vi "Compra.vi"(8 "error in (no error)":errorcluster, 10 "Producto":string[](array[string]), 11 "UI Actor in":refnum<class "UI Actor.lvclass">) -> (0 "error out":errorcluster, 3 "UI Actor out":refnum<class "UI Actor.lvclass">)   [LabVIEW 2019, in "UI Actor.lvlib" / "UI Actor.lvclass"]
uses:
  UI Actor.lvclass
  C:/Program Files/National Instruments/LabVIEW 2019/vi.lib/ActorFramework/Actor/Actor.lvclass
  <vilib>/ActorFramework/Actor/Actor.lvclass/Actor.ctl
  <vilib>/ActorFramework/Message Enqueuer/Message Enqueuer.lvclass/Message Enqueuer.ctl
  UI Actor.lvclass/UI Actor.ctl
  UI Actor Messages/Credit Update Coins Msg/Credit Update Coins Msg.lvclass/Credit Update Coins Msg.ctl
  <vilib>/ActorFramework/Message Enqueuer/Init from Existing Queue.vi
  <vilib>/ActorFramework/Message Enqueuer/Enqueue.vi
  UI Actor Messages/Credit Update Coins Msg/Credit Update Coins Msg.lvclass
  C:/Program Files/National Instruments/LabVIEW 2019/vi.lib/ActorFramework/Message/Message.lvclass
  <vilib>/ActorFramework/Message Priority Queue/Priority Enqueue.vi
  <vilib>/ActorFramework/Message Enqueuer/Message Enqueuer.lvclass
  <vilib>/ActorFramework/Actor/Actor.lvclass
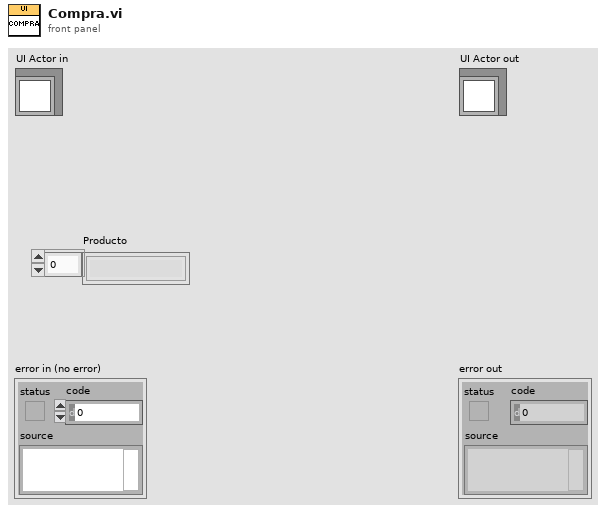
[diagram p1: front panel]
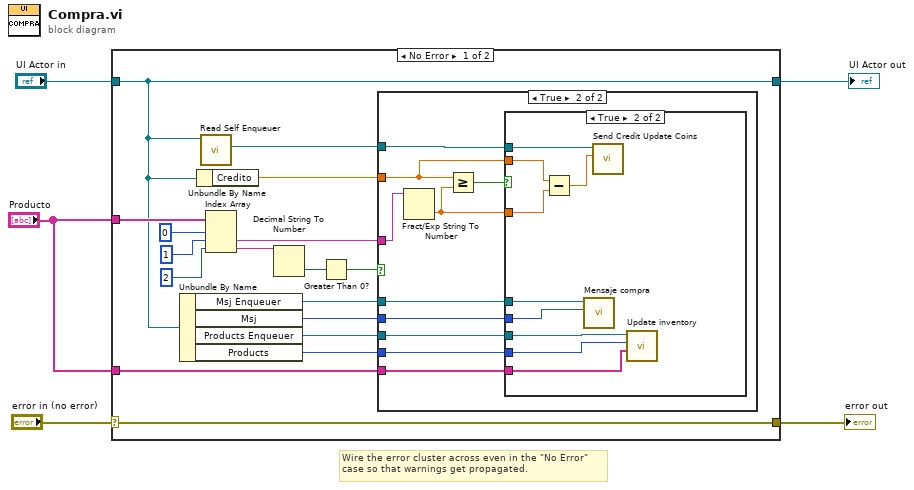
[diagram p0: block diagram]
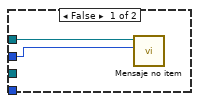
[diagram p2: hidden frame]
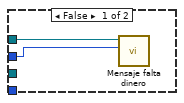
[diagram p3: hidden frame]
diagram:
  # "Wire the error cluster across even in the \"No Error\"\ncase so that warnings get propagated."
  n1 = case shown="No Error" "error in (no error)" {
    selector: "error in (no error)" -> [w22 w47]
    tunnel: [w22 w47] -> w4
    tunnel: [w8 w46] -> w2
    tunnel: "UI Actor in" -> [w8 w46]
    tunnel: "Producto" -> [w21 _]
    tunnel: "Producto" -> [w12 _]
    frame No Error {
      n2 = Unbundle By Name(w8) -> ("Msj Enqueuer"=w6:refnum<class "Message Enqueuer.lvclass">, "Msj"=w7:enum16{"ESP", "ING"}, "Products Enqueuer"=w10:refnum<class "Message Enqueuer.lvclass">, "Products"=w11:enum16{"Bakery", "Coffee"})
      n3 = Unbundle By Name(w8) -> ("Credito"=w14:dbl)
      n4 = call <vilib>:"Read Self Enqueuer.vi"("Actor"=w8) -> ("Self Enqueuer"=w9:refnum<class "Message Enqueuer.lvclass">)  [unwired: 10 in]
      n5 = Index Array(array=w21, index #1=0 ("index"), index #2=1 ("index"), index #3=2 ("index")) -> (element #2=w13:string, element #3=w17:string)  [unwired: 1 out]
      n6 = Decimal String To Number(string=w17) -> (number=w16:i32)  [unwired: 2 in, 1 out]
      n7 = Greater Than 0?(x=w16) -> (x > 0?=w15:bool)
      n8 = case shown="True" w15 {
        tunnel: w14 -> [_ w29]
        tunnel: w13 -> [_ w34]
        tunnel: w12 -> [_ w32]
        tunnel: w11 -> [_ w31]
        tunnel: w10 -> [_ w30]
        tunnel: w9 -> [_ w27]
        tunnel: w7 -> [w24 w26]
        tunnel: w6 -> [w23 w25]
        frame False {
          n9 = call "Mensaje no item.vi"("Msj"=w24, "Message Enqueuer in"=w23) -> ()  [unwired: 10 in]
        }
        frame True {
          n10 = Fract/Exp String To Number(string=w34) -> (number=w28:dbl)  [unwired: 3 in, 1 out]
          n11 = Greater Or Equal?(x=w29, y=w28) -> (x >= y?=w33:bool)
          n12 = case shown="True" w33 {
            tunnel: w32 -> [_ w45]
            tunnel: w31 -> [_ w44]
            tunnel: w30 -> [_ w43]
            tunnel: w29 -> [_ w42]
            tunnel: w28 -> [_ w41]
            tunnel: w27 -> [_ w40]
            tunnel: w26 -> [w36 w38]
            tunnel: w25 -> [w35 w37]
            frame False {
              n13 = call "Mensaje falta dinero.vi"("Msj"=w36, "Message Enqueuer in"=w35) -> ()  [unwired: 10 in]
            }
            frame True {
              n14 = Subtract(x=w42, y=w41) -> (x-y=w39:dbl)
              n15 = call "Mensaje compra.vi"("Msj"=w38, "Message Enqueuer in"=w37) -> ()  [unwired: 10 in]
              n16 = call "Send Credit Update Coins.vi"("Credito"=w39, "Message Enqueuer"=w40) -> ()  [unwired: 8 in, 2 out]
              n17 = call "Update inventory.vi"("Producto"=w45, "Products"=w44, "Message Enqueuer in"=w43) -> ()  [unwired: 9 in]
            }
          }
        }
      }
    }
    frame Error {
    }
  }
  "error out" <- w4
  "UI Actor out" <- w2
